vi "Close.vi"(8 "error in (no error)":errorcluster, 11 "Session Handle":refnum<k15>) -> (0 "error out":errorcluster)   [LabVIEW 2026, in "PXI4072.lvlib"]
uses:
  PXI4072.lvlib
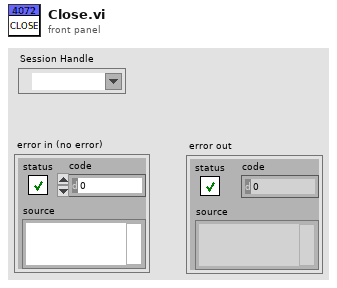
[diagram p1: front panel]
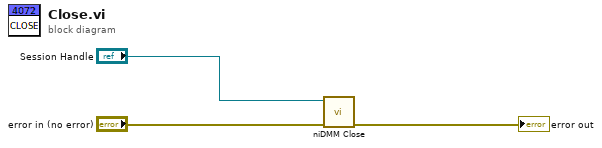
[diagram p0: block diagram]
diagram:
  n1 = call <instrlib>:"niDMM Close.vi"("error in (no error)"="error in (no error)", "instrument handle"="Session Handle") -> ("error out"=→"error out":errorcluster)  [unwired: 9 in]
